vi "Data Measure Current and Voltage.vi"(0 "VISA resource name":refnum<visa-resource-name>, 5 "Channel 1-8 (0:Ch1)":u8(ring) items=["Channel 1", "Channel 2", "Channel 3", "Channel 4", "Channel 5", "Channel 6", "Channel 7", "Channel 8 "], 7 "Input Port (F: Load)":bool, 11 "error in (no error)":errorcluster) -> (4 "VISA resource name out":refnum<visa-resource-name>, 6 "Voltage (V)":dbl format="%.3f", 8 "Current (A)":dbl format="%.3f", 15 "error out":errorcluster)   [LabVIEW 2015, in "Chroma ATE 6310.lvlib"]
doc: "Return current and voltage measured at the input of the electronic load.And you can select the input port of the electronic load to measure voltage."
uses:
  <instrlib>/Chroma ATE 6310/Chroma ATE 6310.lvlib
panel:
  # "UUT\nLoad"
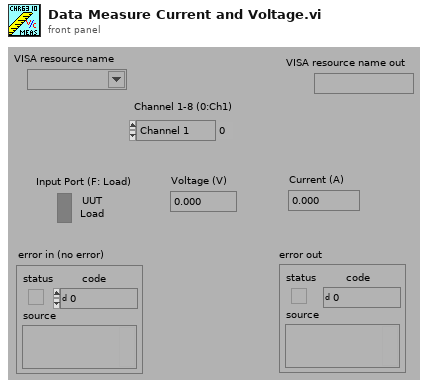
[diagram p1: front panel]
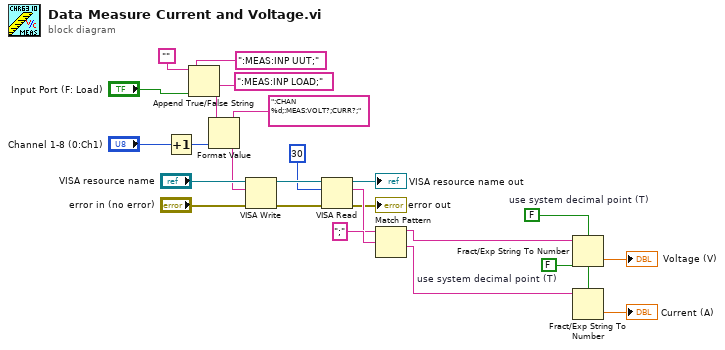
[diagram p0: block diagram]
diagram:
  w1 = FALSE  # use system decimal point (T)
  w2 = FALSE  # use system decimal point (T)
  n1 = Increment(x="Channel 1-8 (0:Ch1)") -> (x+1=w14:u8)
  n2 = Append True/False String(1:"Input Port (F: Load)", 2:":MEAS:INP LOAD;", 3:":MEAS:INP UUT;", 4:"") -> (0:w4:string)
  n3 = Format Value(string ("")=w4, format string=":CHAN %d;:MEAS:VOLT?;CURR?;", value (0)=w14) -> (output string=w8:string)
  n4 = VISA Write(VISA resource name="VISA resource name", write buffer=w8, error in (no error)="error in (no error)") -> (VISA resource name out=w18:refnum<visa-resource-name>, error out=w19:errorcluster)  [unwired: 1 out]
  n5 = VISA Read(VISA resource name=w18, byte count=u32 30, error in (no error)=w19) -> (VISA resource name out=→"VISA resource name out":refnum<visa-resource-name>, read buffer=w15:string, error out=→"error out":errorcluster)  [unwired: 1 out]
  n6 = Match Pattern(string=w15, regular expression=";") -> (before substring=w16:string, after substring=w24:string)  [unwired: 1 in, 2 out]
  n7 = Fract/Exp String To Number(use system decimal point (T)=w1, string=w16) -> (number=→"Voltage (V)":dbl)  [unwired: 2 in, 1 out]
  n8 = Fract/Exp String To Number(use system decimal point (T)=w2, string=w24) -> (number=→"Current (A)":dbl)  [unwired: 2 in, 1 out]
